vi "cast_w12_to_32_bit.vi"(8 "input valid":bool=TRUE, 10 "Shift":i32, 11 "x":fxp<+/-,64,48>) -> (0 "output valid":bool, 3 "y":fxp<+/-,32,14>)   [LabVIEW 2018]
uses:
  <vilib>/rvi/FXPMathLib/FxpConvert/subVIs/nifxpmath_Convert_SimConfig.ctl
  <vilib>/fxp/LVFixedPointQuantizationPolicyTypeDef.ctl
  <vilib>/fxp/LVFixedPointOverflowPolicyTypeDef.ctl
  <vilib>/rvi/FXPMathLib/FxpConvert/simVIs/DllFxpConvertTemp_sub.vi
  <vilib>/rvi/FXPMathLib/FxpInterpret/XNode/nifxpmath_Interpret.xnode
  <vilib>/rvi/FXPMathLib/FxpConvert/XNode/nifxpmath_Convert.xnode
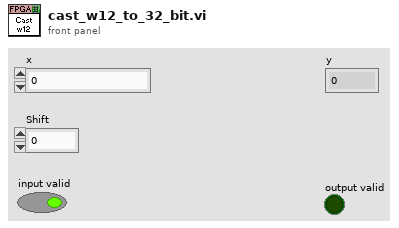
[diagram p1: front panel]
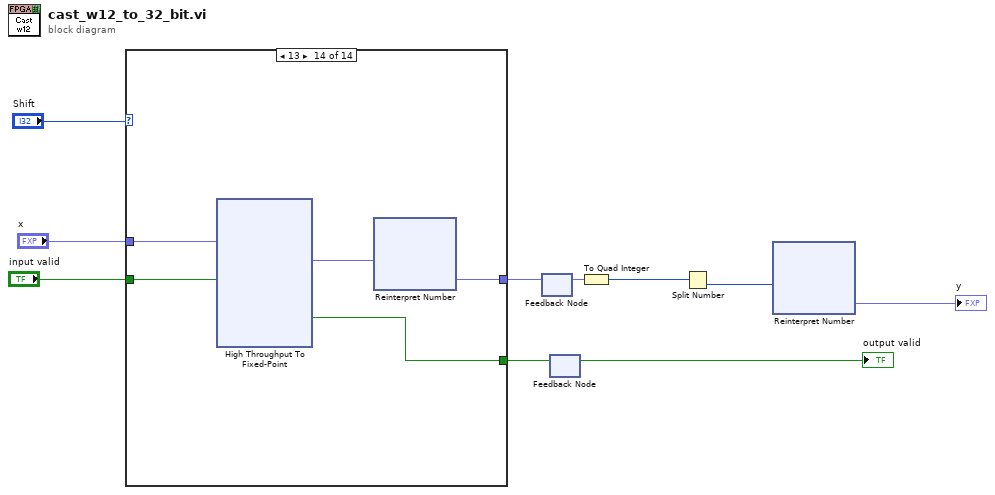
[diagram p0: block diagram]
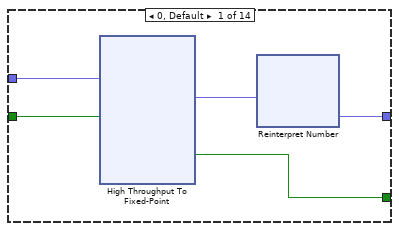
[diagram p2: hidden frame]
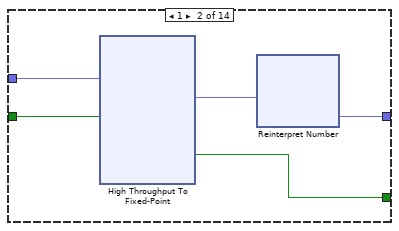
[diagram p3: hidden frame]
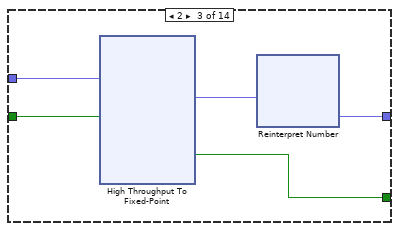
[diagram p4: hidden frame]
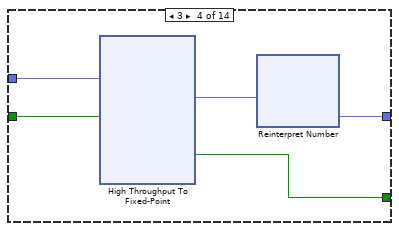
[diagram p5: hidden frame]
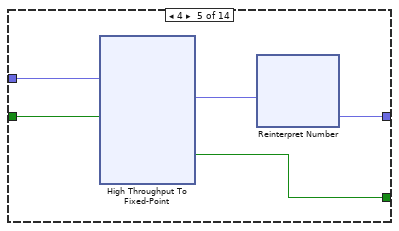
[diagram p6: hidden frame]
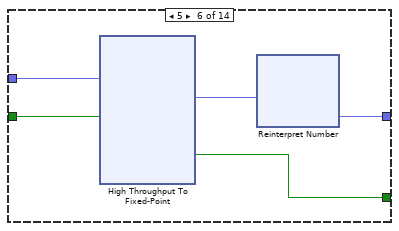
[diagram p7: hidden frame]
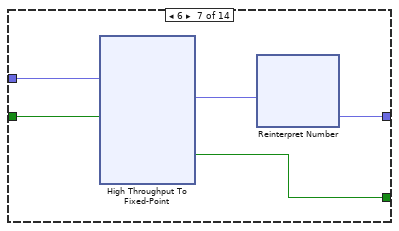
[diagram p8: hidden frame]
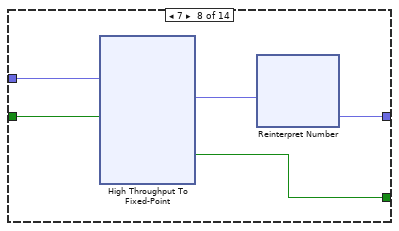
[diagram p9: hidden frame]
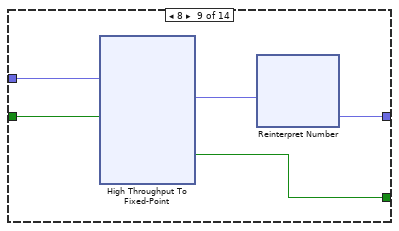
[diagram p10: hidden frame]
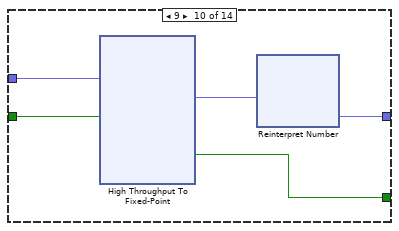
[diagram p11: hidden frame]
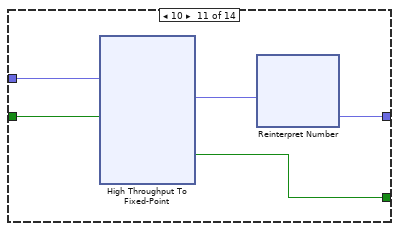
[diagram p12: hidden frame]
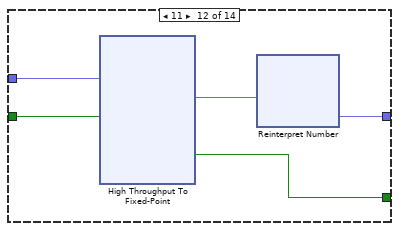
[diagram p13: hidden frame]
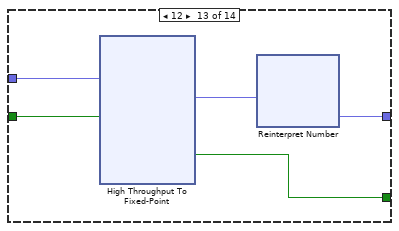
[diagram p14: hidden frame]
diagram:
  n1 = case shown="13" "Shift" {
    tunnel: "x" -> [w15 w44 w73 w102 w131 w160 w189 w218 w247 w276 w305 w334 w363 w392]
    tunnel: [w13 w42 w71 w100 w129 w158 w187 w216 w245 w274 w303 w332 w361 w390] -> w8
    tunnel: "input valid" -> [w12 w41 w70 w99 w128 w157 w186 w215 w244 w273 w302 w331 w360 w389]
    tunnel: [w11 w40 w69 w98 w127 w156 w185 w214 w243 w272 w301 w330 w359 w388] -> w3
    frame 0, Default {
      n2 = xnode "High Throughput To Fixed-Point"("x"=w15, "input valid"=w12) -> ("y"=w14:fxp<+/-,64,49>, "output valid"=w11:bool)  [unwired: 1 in, 1 out]
      n3 = xnode "Reinterpret Number"("x"=w14) -> ("y"=w13:fxp<+/-,64,64>)
    }
    frame 1 {
      n4 = xnode "High Throughput To Fixed-Point"("x"=w44, "input valid"=w41) -> ("y"=w43:fxp<+/-,64,50>, "output valid"=w40:bool)  [unwired: 1 in, 1 out]
      n5 = xnode "Reinterpret Number"("x"=w43) -> ("y"=w42:fxp<+/-,64,64>)
    }
    frame 2 {
      n6 = xnode "High Throughput To Fixed-Point"("x"=w73, "input valid"=w70) -> ("y"=w72:fxp<+/-,64,51>, "output valid"=w69:bool)  [unwired: 1 in, 1 out]
      n7 = xnode "Reinterpret Number"("x"=w72) -> ("y"=w71:fxp<+/-,64,64>)
    }
    frame 3 {
      n8 = xnode "High Throughput To Fixed-Point"("x"=w102, "input valid"=w99) -> ("y"=w101:fxp<+/-,64,52>, "output valid"=w98:bool)  [unwired: 1 in, 1 out]
      n9 = xnode "Reinterpret Number"("x"=w101) -> ("y"=w100:fxp<+/-,64,64>)
    }
    frame 4 {
      n10 = xnode "High Throughput To Fixed-Point"("x"=w131, "input valid"=w128) -> ("y"=w130:fxp<+/-,64,53>, "output valid"=w127:bool)  [unwired: 1 in, 1 out]
      n11 = xnode "Reinterpret Number"("x"=w130) -> ("y"=w129:fxp<+/-,64,64>)
    }
    frame 5 {
      n12 = xnode "High Throughput To Fixed-Point"("x"=w160, "input valid"=w157) -> ("y"=w159:fxp<+/-,64,54>, "output valid"=w156:bool)  [unwired: 1 in, 1 out]
      n13 = xnode "Reinterpret Number"("x"=w159) -> ("y"=w158:fxp<+/-,64,64>)
    }
    frame 6 {
      n14 = xnode "High Throughput To Fixed-Point"("x"=w189, "input valid"=w186) -> ("y"=w188:fxp<+/-,64,55>, "output valid"=w185:bool)  [unwired: 1 in, 1 out]
      n15 = xnode "Reinterpret Number"("x"=w188) -> ("y"=w187:fxp<+/-,64,64>)
    }
    frame 7 {
      n16 = xnode "High Throughput To Fixed-Point"("x"=w218, "input valid"=w215) -> ("y"=w217:fxp<+/-,64,56>, "output valid"=w214:bool)  [unwired: 1 in, 1 out]
      n17 = xnode "Reinterpret Number"("x"=w217) -> ("y"=w216:fxp<+/-,64,64>)
    }
    frame 8 {
      n18 = xnode "High Throughput To Fixed-Point"("x"=w247, "input valid"=w244) -> ("y"=w246:fxp<+/-,64,57>, "output valid"=w243:bool)  [unwired: 1 in, 1 out]
      n19 = xnode "Reinterpret Number"("x"=w246) -> ("y"=w245:fxp<+/-,64,64>)
    }
    frame 9 {
      n20 = xnode "High Throughput To Fixed-Point"("x"=w276, "input valid"=w273) -> ("y"=w275:fxp<+/-,64,58>, "output valid"=w272:bool)  [unwired: 1 in, 1 out]
      n21 = xnode "Reinterpret Number"("x"=w275) -> ("y"=w274:fxp<+/-,64,64>)
    }
    frame 10 {
      n22 = xnode "High Throughput To Fixed-Point"("x"=w305, "input valid"=w302) -> ("y"=w304:fxp<+/-,64,59>, "output valid"=w301:bool)  [unwired: 1 in, 1 out]
      n23 = xnode "Reinterpret Number"("x"=w304) -> ("y"=w303:fxp<+/-,64,64>)
    }
    frame 11 {
      n24 = xnode "High Throughput To Fixed-Point"("x"=w334, "input valid"=w331) -> ("y"=w333:fxp<+/-,64,60>, "output valid"=w330:bool)  [unwired: 1 in, 1 out]
      n25 = xnode "Reinterpret Number"("x"=w333) -> ("y"=w332:fxp<+/-,64,64>)
    }
    frame 12 {
      n26 = xnode "High Throughput To Fixed-Point"("x"=w363, "input valid"=w360) -> ("y"=w362:fxp<+/-,64,61>, "output valid"=w359:bool)  [unwired: 1 in, 1 out]
      n27 = xnode "Reinterpret Number"("x"=w362) -> ("y"=w361:fxp<+/-,64,64>)
    }
    frame 13 {
      n28 = xnode "High Throughput To Fixed-Point"("x"=w392, "input valid"=w389) -> ("y"=w391:fxp<+/-,64,62>, "output valid"=w388:bool)  [unwired: 1 in, 1 out]
      n29 = xnode "Reinterpret Number"("x"=w391) -> ("y"=w390:fxp<+/-,64,64>)
    }
  }
  n30 = feedback #1() -> (w5:fxp<+/-,64,64>)  [unwired: 1 in]
  n31 = feedback-in #1(w8) -> ()
  n32 = feedback #2() -> (→"output valid":bool)  [unwired: 1 in]
  n33 = feedback-in #2(w3) -> ()
  n34 = To Quad Integer(1:w5) -> (0:w9:i64)
  n35 = Split Number(x=w9) -> (lo(x)=w7:u32)  [unwired: 1 out]
  n36 = xnode "Reinterpret Number"("x"=w7) -> ("y"=→"y":fxp<+/-,32,14>)
